vi "Test.vi"() -> ()   [LabVIEW 2012]
uses:
  FIFO(DBL)/FIFO(DBL).lvclass
panel:
  out "Current Size":i32
  out "Current Elements":dbl[](array[numeric])
  out "Removed Element":dbl
  in  "停止":bool
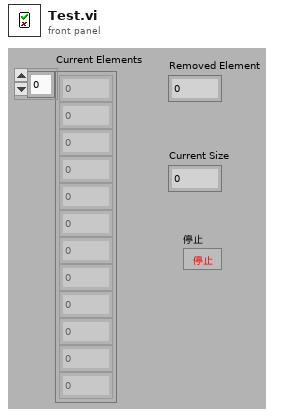
[diagram p1: front panel]
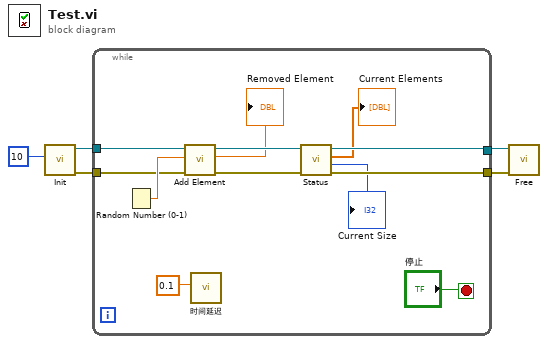
[diagram p0: block diagram]
diagram:
  n1 = call "Init.vi"("size"=10) -> ("error out"=w3:errorcluster, "FIFO(DBL) 输出"=w4:refnum<class "FIFO(DBL).lvclass">)  [unwired: 9 in]
  n2 = while {
    tunnel: w4 -> [w14]
    tunnel: w3 -> [w13]
    tunnel: [w9] -> w2
    tunnel: [w8] -> w1
    stop <- "停止" stop-if-true
    n3 = Random Number (0-1)() -> (number: 0 to 1=w15:dbl)
    n4 = call "Add Element.vi"("error in (no error)"=w13, "Element"=w15, "FIFO(DBL) 输入"=w14) -> ("error out"=w11:errorcluster, "Removed Element"=→"Removed Element":dbl, "FIFO(DBL) 输出"=w12:refnum<class "FIFO(DBL).lvclass">)  [unwired: 6 in]
    n5 = call "时间延迟"("Delay Time (s)"=0.1) -> ()  [unwired: 10 in, 1 out]
    n6 = call "Status.vi"("error in (no error)"=w11, "FIFO(DBL) 输入"=w12) -> ("error out"=w8:errorcluster, "Current Size"=→"Current Size":i32, "Current Elements"=→"Current Elements":dbl[], "FIFO(DBL) 输出"=w9:refnum<class "FIFO(DBL).lvclass">)  [unwired: 6 in]
  }
  n7 = call "Free.vi"("error in (no error)"=w1, "FIFO(DBL) 输入"=w2) -> ()  [unwired: 9 in, 1 out]
